vi "Scan_Barcode.vi"() -> ()   [LabVIEW 2020]
uses:
  <vilib>/userDefined/High Color/IMAQdx.ctl
  <vilib>/vision/driver/NI_Vision_Acquisition_Software.lvlib
  <vilib>/vision/NI_Vision_Development_Module.lvlib
panel:
  in  "stop":bool
  in  "Boolean":bool
  out "ROI Item2":T1 {"Contours"."Type" items=["No Selection", "Point", "Line", "Rectangle", "Oval", "Polygon", "Freehand Region", "Annulus", "Unused2", "Unused3", "Broken Line", "Freehand Line", "Rotated Rectangle"]}
  out "ROI Item1":T1 {"Contours"."Type" items=["No Selection", "Point", "Line", "Rectangle", "Oval", "Polygon", "Freehand Region", "Annulus", "Unused2", "Unused3", "Broken Line", "Freehand Line", "Rotated Rectangle"]}
  in  "Tab Control":enum32{"Position 1", "Position 2", "Position 3"}(tab)
  in  "Data Input":string
  in  "Area1":bool
  in  "Item1":bool
  in  "Area2":bool
  in  "Item2":bool
  in  "Calibration":bool
  in  "Real Data":dbl
  in  "START":bool
  out "Barcode (0) data":string
  out "Result":bool
  out "Image":T2(plugin-control)
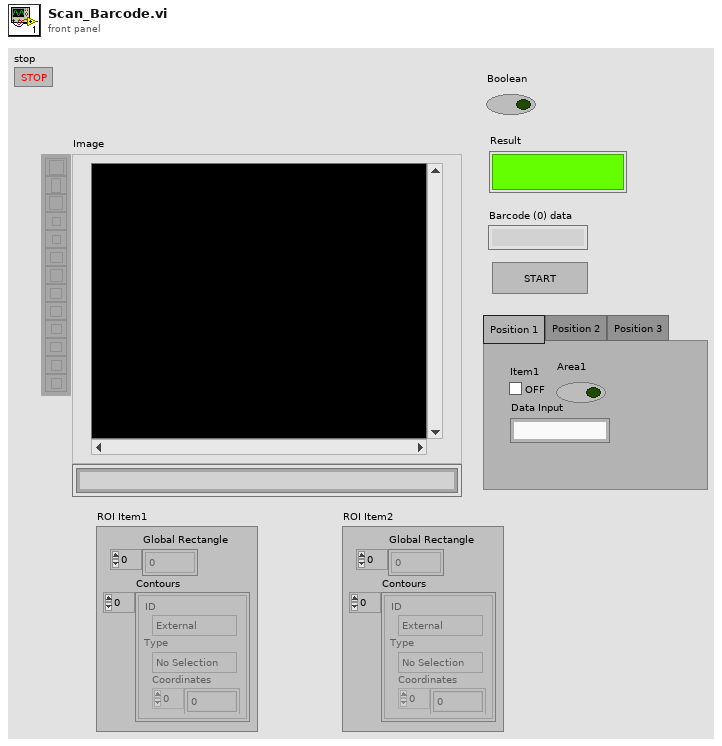
[diagram p1: front panel]
types:
  T1 = typedef "ROI Descriptor" = cluster{"Global Rectangle":i32[], "Contours":cluster{"ID":enum32{"External", "Internal"}, "Type":u32, "Coordinates":i32[]}[]}
  T2 = typedef "IMAQ Image.ctl" = refnum<image>
  T3 = typedef "Image Type" = u32
  T4 = typedef "IMAQdx.ctl" = refnum<k21>
  T5 = cluster{"Global Rectangle":i32[], "Contours":cluster{"Contour Type":u32, "ROI Type":u32, "Points":i32[]}[]}
  T6 = cluster{"Data":string, "Special Char 1":string, "Special Char 2":string, "Checksum(s)":string, "Barcode Type":u32, "Confidence Level":sgl, "Bounding Box":cluster{"x":sgl, "y":sgl}[]}[]
  T7 = cluster{"Barcodes[0]":cluster{"Data":string, "Special Char 1":string, "Special Char 2":string, "Checksum(s)":string, "Barcode Type":u32, "Confidence Level":sgl, "Bounding Box":cluster{"x":sgl, "y":sgl}[]}, "Barcodes[1]":cluster{"Data":string, "Special Char 1":string, "Special Char 2":string, "Checksum(s)":string, "Barcode Type":u32, "Confidence Level":sgl, "Bounding Box":cluster{"x":sgl, "y":sgl}[]}, "Barcodes[2]":cluster{"Data":string, "Special Char 1":string, "Special Char 2":string, "Checksum(s)":string, "Barcode Type":u32, "Confidence Level":sgl, "Bounding Box":cluster{"x":sgl, "y":sgl}[]}, "Barcodes[3]":cluster{"Data":string, "Special Char 1":string, "Special Char 2":string, "Checksum(s)":string, "Barcode Type":u32, "Confidence Level":sgl, "Bounding Box":cluster{"x":sgl, "y":sgl}[]}, "Barcodes[4]":cluster{"Data":string, "Special Char 1":string, "Special Char 2":string, "Checksum(s)":string, "Barcode Type":u32, "Confidence Level":sgl, "Bounding Box":cluster{"x":sgl, "y":sgl}[]}, "Barcodes[5]":cluster{"Data":string, "Special Char 1":string, "Special Char 2":string, "Checksum(s)":string, "Barcode Type":u32, "Confidence Level":sgl, "Bounding Box":cluster{"x":sgl, "y":sgl}[]}, "Barcodes[6]":cluster{"Data":string, "Special Char 1":string, "Special Char 2":string, "Checksum(s)":string, "Barcode Type":u32, "Confidence Level":sgl, "Bounding Box":cluster{"x":sgl, "y":sgl}[]}, "Barcodes[7]":cluster{"Data":string, "Special Char 1":string, "Special Char 2":string, "Checksum(s)":string, "Barcode Type":u32, "Confidence Level":sgl, "Bounding Box":cluster{"x":sgl, "y":sgl}[]}, "Barcodes[8]":cluster{"Data":string, "Special Char 1":string, "Special Char 2":string, "Checksum(s)":string, "Barcode Type":u32, "Confidence Level":sgl, "Bounding Box":cluster{"x":sgl, "y":sgl}[]}}
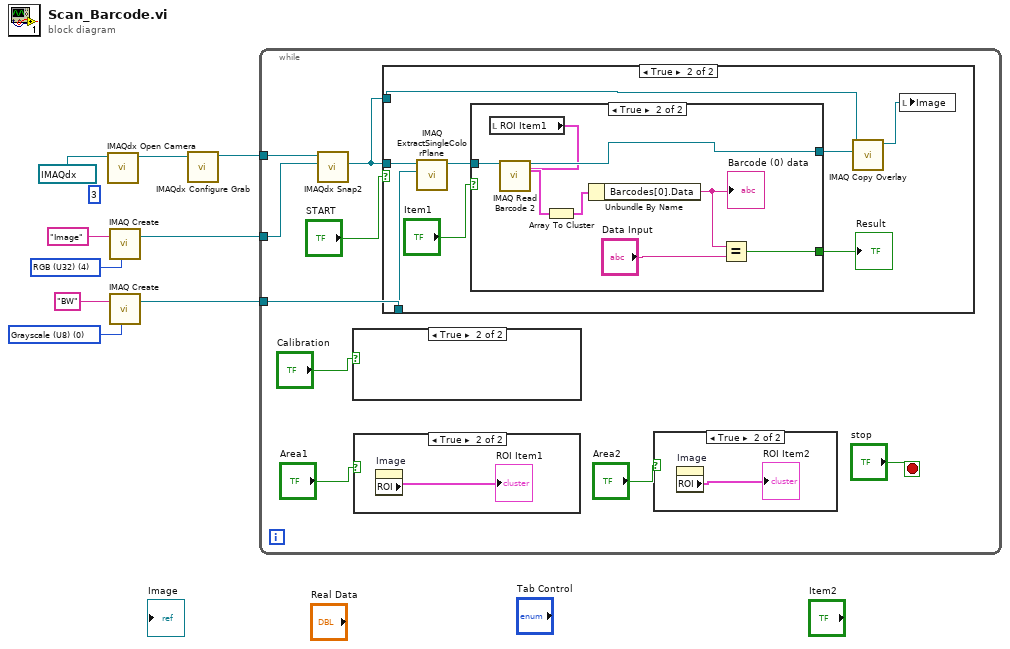
[diagram p0: block diagram]
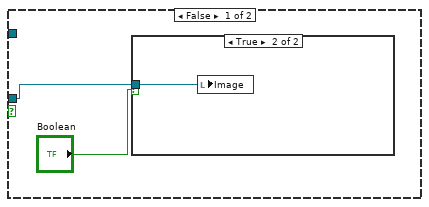
[diagram p5: hidden frame]
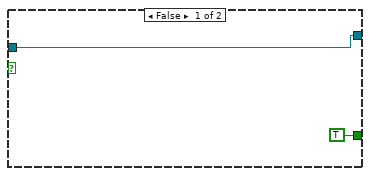
[diagram p7: hidden frame]
diagram:
  w2 = T3 0 items=["Grayscale (U8)", "Grayscale (I16)", "Grayscale (SGL)", "Complex (CSG)", "RGB (U32)", "HSL (U32)", "RGB (U64)", "Grayscale (U16)"] ("Image Type")
  w7 = T3 4 items=["Grayscale (U8)", "Grayscale (I16)", "Grayscale (SGL)", "Complex (CSG)", "RGB (U32)", "HSL (U32)", "RGB (U64)", "Grayscale (U16)"] ("Image Type")
  (unwired) 3 ("Border Size")
  n1 = call <vilib>:"IMAQdx Open Camera.vi"("Session In"=T4 "cam5") -> ("Session Out"=w6:T4)  [unwired: 9 in, 1 out]
  n2 = call "IMAQ Create"("Image Name"="Image", "Image Type"=w7) -> ("New Image"=w4:T2)  [unwired: 3 in, 1 out]
  n3 = call "IMAQ Create"("Image Name"="BW", "Image Type"=w2) -> ("New Image"=w1:T2)  [unwired: 3 in, 1 out]
  n4 = call <vilib>:"IMAQdx Configure Grab.vi"("Session In"=w6) -> ("Session Out"=w5:T4)  [unwired: 9 in, 1 out]
  n5 = while {
    tunnel: w5 -> [w17]
    tunnel: w4 -> [w16]
    tunnel: w1 -> [w15]
    stop <- "stop" stop-if-true
    n6 = call <vilib>:"IMAQdx Snap2.vi"("Image In"=w16, "Session In"=w17) -> ("Image Out"=w13:T2)  [unwired: 7 in, 2 out]
    n7 = case shown="True" "Calibration" {
      frame False {
      }
      frame True {
      }
    }
    n8 = case shown="True" "Area1" {
      frame False {
      }
      frame True {
        n9 = property on="Image" class="ImageControl"() -> ("ROI"=→"ROI Item1":T5)  [unwired: 2 in, 2 out]
      }
    }
    n10 = case shown="True" "START" {
      tunnel: w15 -> [_ w31]
      tunnel: w13 -> [w22 w29]
      tunnel: w13 -> [_ w27]
      frame False {
        n11 = case shown="True" "Boolean" {
          tunnel: w22 -> [_ w23]
          frame False {
          }
          frame True {
            n12 = local write "Image"(w23) -> ()
          }
        }
      }
      frame True {
        n13 = call "IMAQ ExtractSingleColorPlane"("Image Dst"=w31, "Image Src"=w29) -> ("Image Dst Out"=w28:T2)  [unwired: 8 in, 1 out]
        n14 = case shown="True" "Item1" {
          tunnel: w28 -> [w33 w41]
          tunnel: [w33 w38] -> w26
          tunnel: [TRUE w34] -> w25
          frame False {
          }
          frame True {
            n15 = local read "ROI Item1"() -> (w37:T1)
            n16 = call "IMAQ Read Barcode 2"("Image"=w41, "ROI Descriptor"=w37) -> ("Image (duplicate)"=w38:T2, "Barcodes"=w40:T6)  [unwired: 9 in, 3 out]
            n17 = Array To Cluster(array=w40) -> (cluster=w39:T7)
            n18 = Unbundle By Name(w39) -> ("Barcodes[0].Data"=w36:string)
            "Barcode (0) data" <- w36
            n19 = Equal?(x=w36, y="Data Input") -> (x = y?=w34:bool)
          }
        }
        "Result" <- w25
        n20 = call "IMAQ Copy Overlay"("Image Dst"=w26, "Image Src"=w27) -> ("Image Dst Out"=w24:T2)  [unwired: 8 in, 1 out]
        n21 = local write "Image"(w24) -> ()
      }
    }
    n22 = case shown="True" "Area2" {
      frame False {
      }
      frame True {
        n23 = property on="Image" class="ImageControl"() -> ("ROI"=→"ROI Item2":T5)  [unwired: 2 in, 2 out]
      }
    }
  }
